vi "GoalieNormal.vi"(6 "atacando contra?":bool=TRUE, 7 "Stop?":bool=TRUE, 8 "Robot":T3={"id"=0, "function"=enum."Attacker", "x"=0.0, "y"=0.0, "orientation"=0.0, "v_tangent"=0.0, "v_normal"=0.0, "v_ang"=0.0, "kick_x"=0.0, "kick_z"=0.0, "dribble"=FALSE, "Timestamp"=timestamp(0 s since 1904-01-01), "estimatives"={"est_v_tangent"=0.0, "est_v_normal"=0.0, "est_vx"=0.0, "est_vy"=0.0, "Pos Robot Est"=[]}, "dest_x_kick"=0.0, "dest_y_kick"=0.0, "Gap Coord"=[], "States"=enum."GoToTangent", "Path "=[], "Path  Smooth"=[], "Dest"=[]}, 9 "AI Parameters":T1={"GotoKick"={"Dist do cone a frente"=150.0, "attacker farback"=1500.0, "Perto"=300.0, "min dist to kick"=150.0, "kick eps"=0.0, "Time to transition"=0.05}, "Attacker"={"CC chute"=0.09, "CC passe"=0.045, "Kick Force"=100.0, "ball-robot Kick"=200.0, "ball-robot Pass"=0.3, "drible\nAttk"=FALSE}, "Defender"={"D max"=1700.0, "Vel p/ robô av"=1000.0, "Kick Force"=100.0, "D atk-def"=0.0, "D farback"=0.0, "drible\ndef"=FALSE, "drible\ngoalie"=FALSE}, "Timeout"={"Field/v in x"=6.0, "Dist Robots"=300, "Dist up in y"=300}, "Pose Striker"={"dist"=200.0, "Numeric"=-4.0, "dist 2"=200.0, "drible\nstriker"=FALSE}, "Dist Stop"=300.0, "D ball out"=200, "D central gap "=150.0, "T pass"=0.0, "Force ++"=0.0, "range kick"=0.0, "Chute alto"=TRUE, "Marcador novo"=TRUE, "drible"=FALSE, "D drible"=300.0} {"D drible" format="%#_13g"; "D central gap" format="%#_13g"; "Dist Stop" format="%#_13g"; "Pose Striker"."Numeric" format="%#_13g"; "Defender"."Kick Force" format="%#_13g"; "Defender"."Vel p/ robô av" format="%#_13g"; "Attacker"."ball-robot Kick" format="%#_13g"; "Attacker"."Kick Force" format="%#_13g"; "Attacker"."CC passe" format="%#_13g"; "Attacker"."CC chute" format="%#_13g"; "GotoKick"."kick eps" format="%#_13g"; "GotoKick"."min dist to kick" format="%#_13g"; "GotoKick"."Perto" format="%#_13g"; "GotoKick"."attacker farback" format="%#_13g"; "GotoKick"."Dist do cone a frente" format="%#_13g"}, 10 "geometry":T2, 11 "IA Input":T8={"our_robots"=[], "enemy_robots"=[], "balls"=[], "geometry"={"line_width"=0, "field_length"=0, "field_width"=0, "boundary_width"=0, "referee_width"=0, "goal_width"=0, "goal_depth"=0, "goal_wall_width"=0, "center_circle_radius"=0, "defense_radius"=0, "defense_stretch"=0, "free_kick_from_defense_dist"=0, "penalty_spot_from_field_line_dist"=0, "penalty_line_from_spot_dist"=0}, "IA Judge"={"stage"="", "command"="", "our_goalie_id"=0.0, "enemy_goalie_id"=0.0, "command enum"=enum."Halt", "Time"=enum."Azul"}, "Received Timestamp"=timestamp(0 s since 1904-01-01), "Events"={"Touch"=FALSE, "Ball out"=FALSE, "id touch"=0.0, "Ball out of \nVision"=FALSE, "Ball inside \nGoalie area"=FALSE, "Robot not responding"=FALSE, "Robots responding status"=[1.0, 1.0, 1.0, 1.0, 1.0, 1.0], "Enemy Ball \nPossession"=FALSE, "Pass State"=FALSE, "id end of pass"=0.0, "Kick"=FALSE, "Id ini Possession"=0.0, "Ball Possesion"=FALSE, "Id Possesion"=0.0}}) -> (3 "output cluster":T3={"id"=0, "function"=enum."Attacker", "x"=0.0, "y"=0.0, "orientation"=0.0, "v_tangent"=0.0, "v_normal"=0.0, "v_ang"=0.0, "kick_x"=0.0, "kick_z"=0.0, "dribble"=FALSE, "Timestamp"=timestamp(0 s since 1904-01-01), "estimatives"={"est_v_tangent"=0.0, "est_v_normal"=0.0, "est_vx"=0.0, "est_vy"=0.0, "Pos Robot Est"=[]}, "dest_x_kick"=0.0, "dest_y_kick"=0.0, "Gap Coord"=[], "States"=enum."GoToTangent", "Path "=[], "Path  Smooth"=[], "Dest"=[]})   [LabVIEW 2017]
uses:
  Core/AI Input.ctl
  Core/AI Robot.ctl
  Functions Enum.ctl
  AttackerStates.ctl
  Path Planning/RRT/PathDests.ctl
  Path Planning/RRT/PathDest.ctl
  Core/AI Ball.ctl
  Core/Field Size.ctl
  Core/AI Judge.ctl
  Command Enum.ctl
  Util/Events/Events.ctl
  AI Parameters.ctl
  PersonalityEnum.ctl
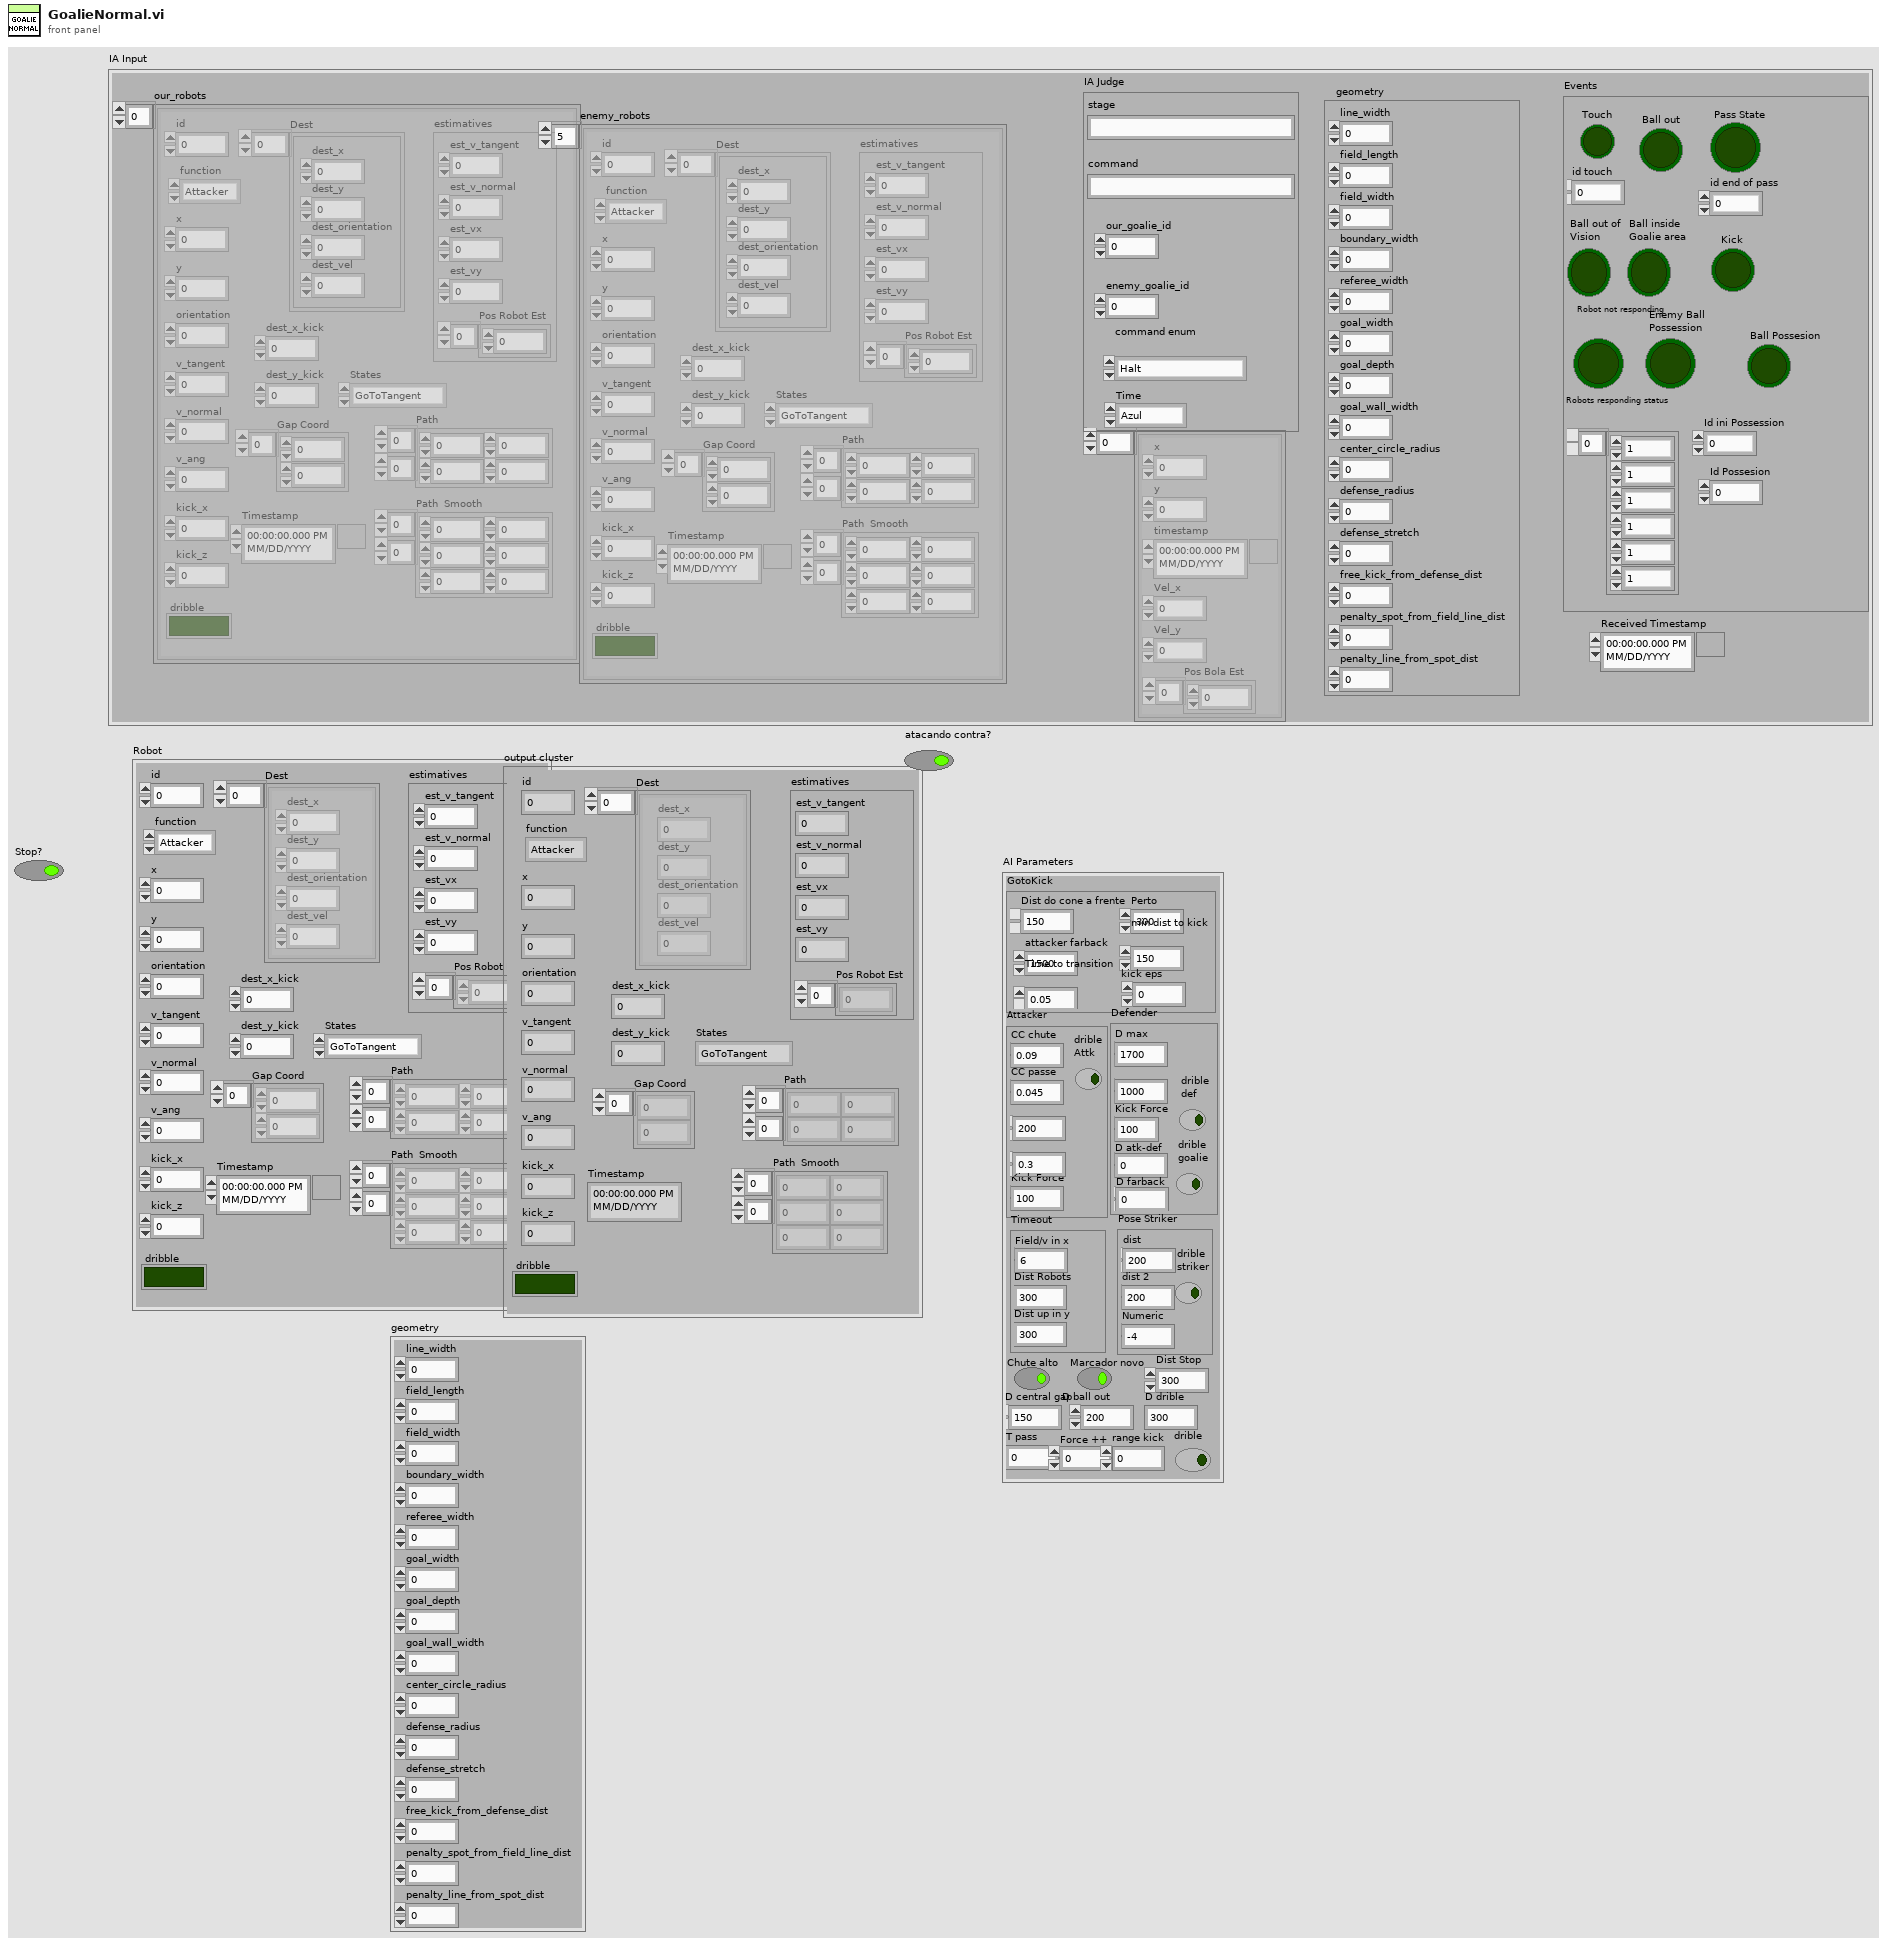
[diagram p1: front panel]
types:
  T1 = typedef "AI Parameters.ctl" = cluster{"GotoKick":cluster{"Dist do cone a frente":dbl, "attacker farback":dbl, "Perto":dbl, "min dist to kick":dbl, "kick eps":dbl, "Time to transition":dbl}, "Attacker":cluster{"CC chute":dbl, "CC passe":dbl, "Kick Force":dbl, "ball-robot Kick":dbl, "ball-robot Pass":dbl, "drible\nAttk":bool}, "Defender":cluster{"D max":dbl, "Vel p/ robô av":dbl, "Kick Force":dbl, "D atk-def":dbl, "D farback":dbl, "drible\ndef":bool, "drible\ngoalie":bool}, "Timeout":cluster{"Field/v in x":dbl, "Dist Robots":u32, "Dist up in y":u32}, "Pose Striker":cluster{"dist":dbl, "Numeric":dbl, "dist 2":dbl, "drible\nstriker":bool}, "Dist Stop":dbl, "D ball out":i32, "D central gap ":dbl, "T pass":dbl, "Force ++":dbl, "range kick":dbl, "Chute alto":bool, "Marcador novo":bool, "drible":bool, "D drible":dbl}
  T2 = typedef "Field Size.ctl" = cluster{"line_width":u32, "field_length":u32, "field_width":u32, "boundary_width":u32, "referee_width":u32, "goal_width":u32, "goal_depth":u32, "goal_wall_width":u32, "center_circle_radius":u32, "defense_radius":u32, "defense_stretch":u32, "free_kick_from_defense_dist":u32, "penalty_spot_from_field_line_dist":u32, "penalty_line_from_spot_dist":u32}
  T3 = typedef "AI Robot.ctl" = cluster{"id":u32, "function":T4, "x":dbl, "y":dbl, "orientation":dbl, "v_tangent":dbl, "v_normal":dbl, "v_ang":dbl, "kick_x":dbl, "kick_z":dbl, "dribble":bool, "Timestamp":timestamp, "estimatives":cluster{"est_v_tangent":dbl, "est_v_normal":dbl, "est_vx":dbl, "est_vy":dbl, "Pos Robot Est":dbl[]}, "dest_x_kick":dbl, "dest_y_kick":dbl, "Gap Coord":dbl[], "States":T5, "Path ":dbl[][], "Path  Smooth":dbl[][], "Dest":T6}
  T4 = typedef "Functions Enum.ctl" = enum16{"Attacker", "Goalie", "Defender", "Striker", "Goto 0", "Dummy", "Kicker", "ZigZag 0", "ZigZag 1", "ZigZag 2", "ZigZag 3", "ZigZag 4", "ZigZag 5", "ZigZag 6", "ZigZag 7", "ZigZag 8", ""}
  T5 = typedef "AttackerStates.ctl" = enum16{"Pass", "GoToTangent", "BallGetting", "GoToKick", ""}
  T6 = typedef "PathDests.ctl" = T7[]
  T7 = typedef "PathDest.ctl" = cluster{"dest_x":dbl, "dest_y":dbl, "dest_orientation":dbl, "dest_vel":dbl}
  T8 = typedef "AI Input.ctl" = cluster{"our_robots":T3[], "enemy_robots":T3[], "balls":T9[], "geometry":T2, "IA Judge":T10, "Received Timestamp":timestamp, "Events":T12}
  T9 = typedef "AI Ball.ctl" = cluster{"x":dbl, "y":dbl, "timestamp":timestamp, "Vel_x":dbl, "Vel_y":dbl, "Pos Bola Est":dbl[]}
  T10 = typedef "AI Judge.ctl" = cluster{"stage":string, "command":string, "our_goalie_id":dbl, "enemy_goalie_id":dbl, "command enum":T11, "Time":enum16{"Azul", "Amarelo"}}
  T11 = typedef "Command Enum.ctl" = enum16{"Halt", "Stop", "Force Start", "PKA Normal Start", "Prepare Kickoff Ally", "PKE Normal Start", "Prepare Kickoff Enemy", "Prepare Penalty Ally", "PPA Normal Start", "Prepare Penalty Enemy", "PPE Normal Start", "Direct Free Enemy", "Direct Free Ally", "Indirect Free Enemy", "Indirect Free Ally", "Timeout Enemy", "Timeout Ally", "Goal Enemy", "Goal Ally", "Ball Placement Enemy", "Ball Placement Ally", "Normal Half Time", "Extra Time Break", "Extra Half Time", "None", "Post Game"}
  T12 = typedef "Events.ctl" = cluster{"Touch":bool, "Ball out":bool, "id touch":dbl, "Ball out of \nVision":bool, "Ball inside \nGoalie area":bool, "Robot not responding":bool, "Robots responding status":dbl[], "Enemy Ball \nPossession":bool, "Pass State":bool, "id end of pass":dbl, "Kick":bool, "Id ini Possession":dbl, "Ball Possesion":bool, "Id Possesion":dbl}
  T13 = typedef "PersonalityEnum.ctl" = enum16{"Attacker", "Striker", "Defender", "Goalie"}
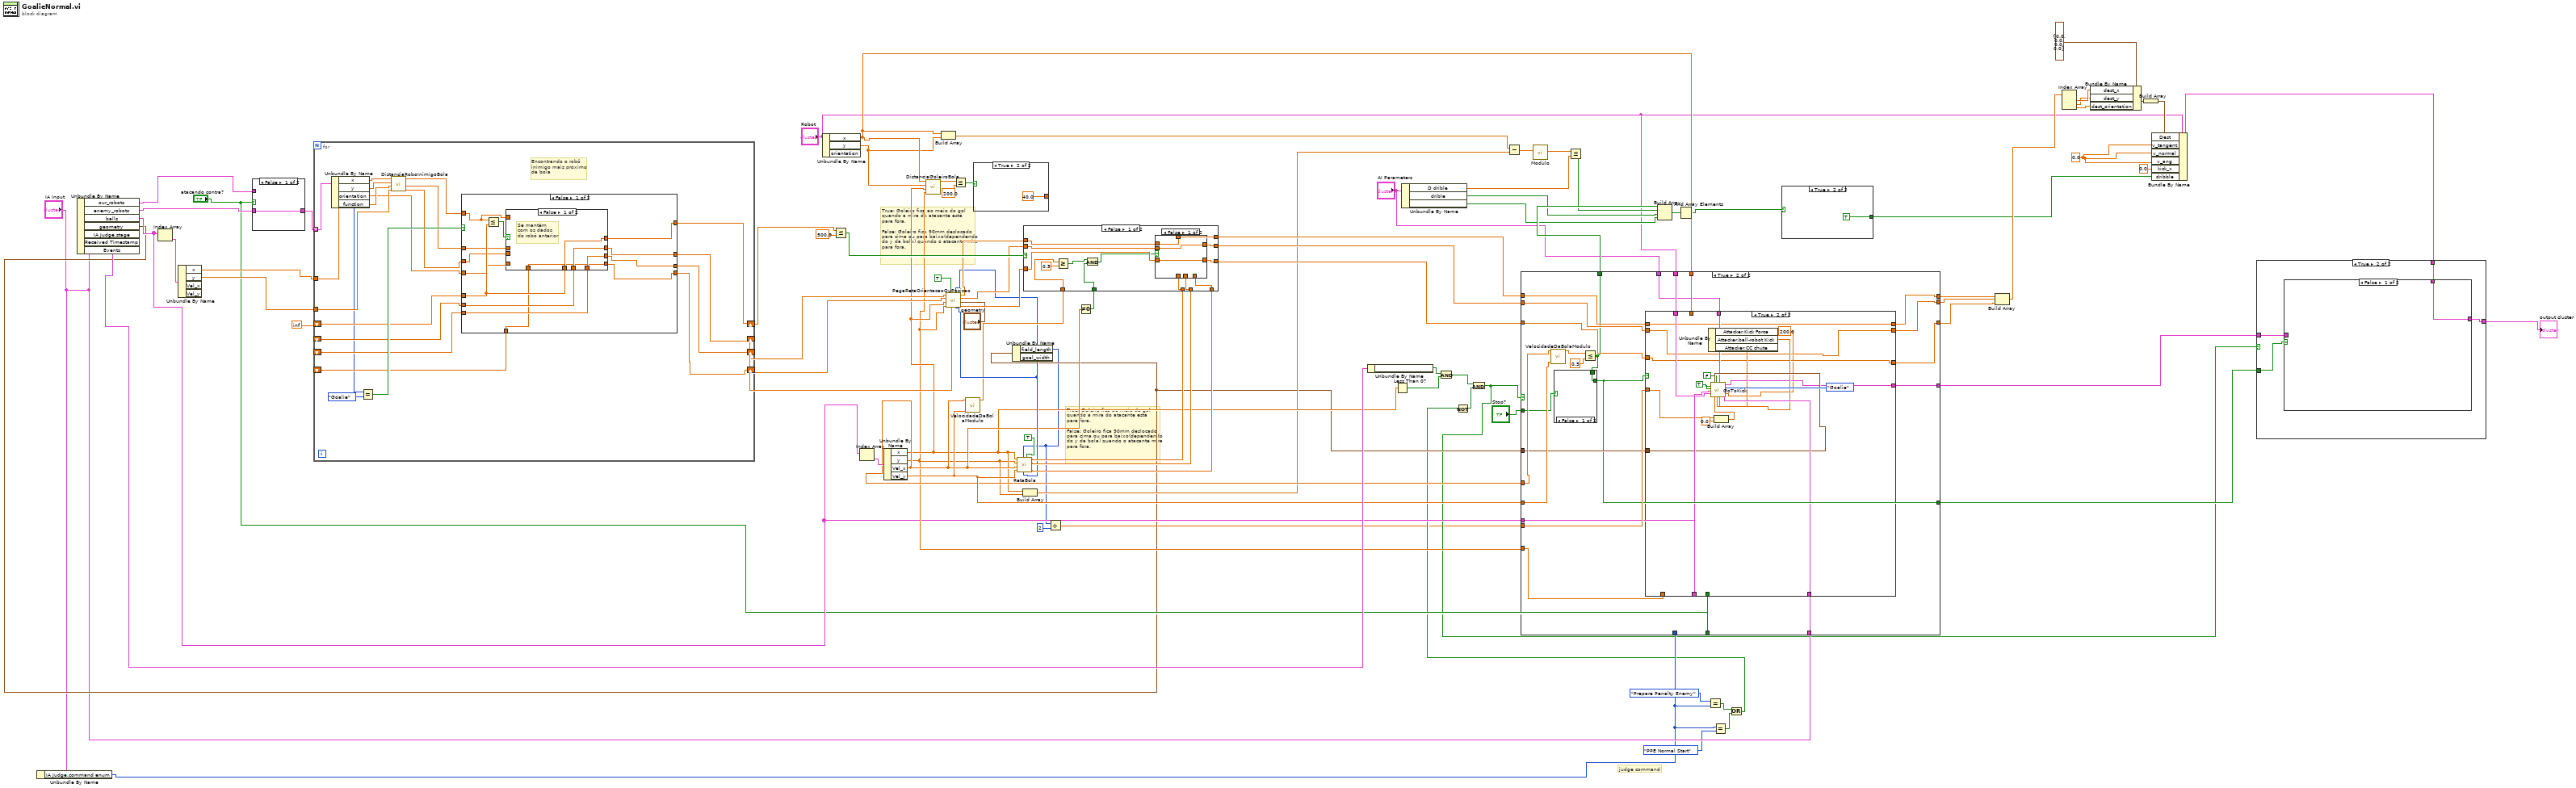
[diagram p0: block diagram]
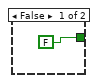
[diagram p4: hidden frame]
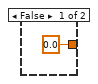
[diagram p6: hidden frame]
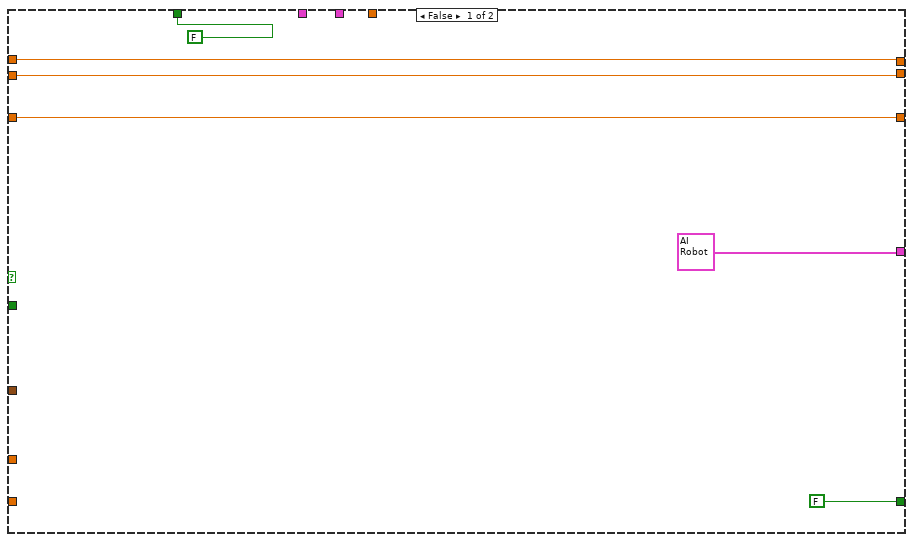
[diagram p7: hidden frame]
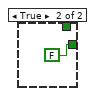
[diagram p8: hidden frame]
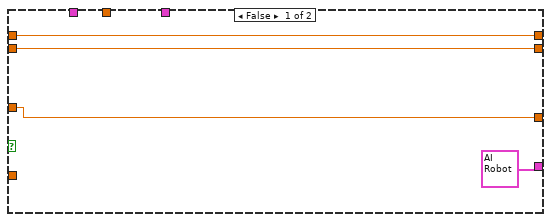
[diagram p9: hidden frame]
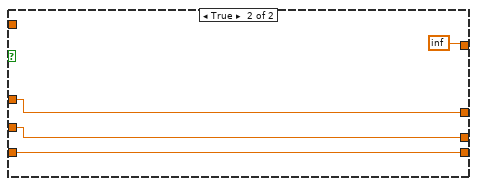
[diagram p13: hidden frame]
diagram:
  w41 = 0.0
  # "judge command"
  # "True: Goleiro fica ao meio do gol\nquando a mira do atacante está\npara fora.\n\nFalse: Goleiro fica 90mm deslocado\npara cima ou para baixo(dependendo\ndo y da bola) quando o atacante mira\npara fora."
  # "True: Goleiro fica ao meio do gol\nquando a mira do atacante está\npara fora.\n\nFalse: Goleiro fica 90mm deslocado\npara cima ou para baixo(dependendo\ndo y da bola) quando o atacante mira\npara fora."
  n1 = Unbundle By Name("IA Input") -> ("IA Judge.command enum"=w10:T11)
  n2 = Unbundle By Name("IA Input") -> ("our_robots"=w64:T3[], "enemy_robots"=w66:T3[], "balls"=w23:T9[], "geometry"=w20:T2, "Events"=w81:T12)  [unwired: 2 out]
  n3 = Index Array(array=w23) -> (element=w88:T9)  [unwired: 1 in]
  n4 = Unbundle By Name(w88) -> ("x"=w87:dbl, "y"=w86:dbl)  [unwired: 2 out]
  n5 = case shown="False" "atacando contra?" {
    tunnel: [w89 w90] -> w65
    tunnel: w66 -> [w89 _]
    tunnel: w64 -> [_ w90]
    frame False {
    }
    frame True {
    }
  }
  n6 = for {
    tunnel: w65 -> [w102] mode=indexing
    tunnel: w87 -> [w107]
    tunnel: w86 -> [w106]
    shift-right: [w104] -> w84
    shift-left: inf -> [w103]
    shift-right: [w100] -> w57
    shift-left: _ -> [w97]
    shift-right: [w98] -> w58
    shift-left: _ -> [w96]
    shift-right: [w94] -> w63
    shift-left: _ -> [w93]
    # "Encontrando o robô \ninimigo mais próximo\nda bola"
    n7 = Unbundle By Name(w102) -> ("x"=w109:dbl, "y"=w108:dbl, "orientation"=w95:dbl, "function"=w92:T4)
    n8 = Equal?(x=w92, y=Functions_Enum."Goalie") -> (x = y?=w110:bool)
    n9 = call "DistanciaRoboInimigoBola.vi"("Y bola"=w106, "X bola"=w107, "Y inimigo"=w108, "X inimigo"=w109) -> ("Y inimigo"=w99:dbl, "X inimigo"=w101:dbl, "Distância"=w105:dbl)  [unwired: 5 in]
    n10 = case shown="False" w110 {
      tunnel: [w122 inf] -> w104
      tunnel: w105 -> [w121 _]
      tunnel: w103 -> [w120 _]
      tunnel: w101 -> [w116 w135]
      tunnel: [w118 w135] -> w100
      tunnel: w99 -> [w115 w134]
      tunnel: [w112 w134] -> w98
      tunnel: w97 -> [w119 _]
      tunnel: w96 -> [w117 _]
      tunnel: w95 -> [w114 w133]
      tunnel: [w113 w133] -> w94
      tunnel: w93 -> [w111 _]
      frame False {
        n11 = Less Or Equal?(x=w121, y=w120) -> (x <= y?=w123:bool)
        n12 = case shown="False" w123 {
          tunnel: [w127 w131] -> w122
          tunnel: w121 -> [_ w131]
          tunnel: w120 -> [w127 _]
          tunnel: w119 -> [w126 _]
          tunnel: [w126 w130] -> w118
          tunnel: w117 -> [w125 _]
          tunnel: [w125 w129] -> w112
          tunnel: w116 -> [_ w130]
          tunnel: w115 -> [_ w129]
          tunnel: w114 -> [_ w128]
          tunnel: [w124 w128] -> w113
          tunnel: w111 -> [w124 _]
          frame False {
            # "Se mantém \ncom os dados\ndo robô anterior"
          }
          frame True {
            # "Fica com os\ndados do robô\natual"
          }
        }
      }
      frame True {
      }
    }
  }
  n13 = Unbundle By Name("Robot") -> ("x"=w40:dbl, "y"=w39:dbl)  [unwired: 1 out]
  n14 = Less Or Equal?(x=w84, y=500.0) -> (x <= y?=w82:bool)
  n15 = Index Array(array=w23) -> (element=w85:T9)  [unwired: 1 in]
  n16 = Unbundle By Name(w85) -> ("x"=w37:dbl, "y"=w36:dbl, "Vel_x"=w52:dbl, "Vel_y"=w53:dbl)
  n17 = call "DistanciaGoleiroBola.vi"("Y bola"=w36, "X bola"=w37, "Y goleiro"=w39, "X goleiro"=w40) -> ("Distância"=w74:dbl)  [unwired: 7 in]
  n18 = Build Array(w40, w39) -> (w38:dbl[])
  n19 = Less Or Equal?(x=w74, y=200.0) -> (x <= y?=w72:bool)
  n20 = call "VelocidadeDaBolaModulo.vi"("Vy bola"=w53, "Vx bola"=w52) -> ("Vel bola"=w54:dbl)  [unwired: 9 in]
  n21 = case shown="True" w72 {
    tunnel: [0.0 40.0] -> _
    frame False {
    }
    frame True {
    }
  }
  n22 = Unbundle By Name(w20) -> ("field_length"=w3:u32, "goal_width"=w62:u32)
  n23 = call "PegaRetaOrientacaoOuPosicao.vi"("Field Size 2"="geometry", "Goal Width"=w62, "Field Length"=w3, "Orientação inimigo"=w63, "Meio?"=TRUE, "Y bola"=w36, "X bola"=w37, "Y inimigo"=w58, "X inimigo"=w57) -> ("Orientação goleiro"=w59:dbl, "Y goleiro"=w60:dbl, "X goleiro"=w61:dbl)
  n24 = call "RetaBola.vi"("Meio?"=TRUE, "Goal Width"=w62, "Field Lenght"=w3, "Vy bola"=w53, "Vx bola"=w52, "Y bola"=w36, "X bola"=w37) -> ("Orientação"=w68:dbl, "Y goleiro"=w69:dbl, "X goleiro"=w70:dbl)  [unwired: 2 in]
  n25 = Build Array(w37, w36) -> (w35:dbl[])
  n26 = Divide(x=w3, y=u32 2) -> (x/y=w2:dbl)
  n27 = Not Equal To 0?(x=w52) -> (x != 0?=w51:bool)
  n28 = case shown="False" w82 {
    tunnel: [w149 w160] -> w80
    tunnel: w61 -> [w143 w160]
    tunnel: [w147 w159] -> w78
    tunnel: w60 -> [w142 w159]
    tunnel: [w144 w158] -> w76
    tunnel: w59 -> [w141 w158]
    tunnel: w70 -> [w148 _]
    tunnel: w69 -> [w146 _]
    tunnel: w68 -> [w145 _]
    tunnel: w54 -> [w150 _]
    tunnel: w51 -> [w139 _]
    frame False {
      n29 = Greater Or Equal?(x=w150, y=0.5) -> (x >= y?=w140:bool)
      n30 = And(x=w140, y=w139) -> (x .and. y?=w138:bool)
      n31 = case shown="False" w138 {
        tunnel: [w154 w157] -> w149
        tunnel: w148 -> [_ w157]
        tunnel: [w153 w156] -> w147
        tunnel: w146 -> [_ w156]
        tunnel: w145 -> [_ w155]
        tunnel: [w152 w155] -> w144
        tunnel: w143 -> [w154 _]
        tunnel: w142 -> [w153 _]
        tunnel: w141 -> [w152 _]
        frame False {
        }
        frame True {
        }
      }
    }
    frame True {
    }
  }
  n32 = Unbundle By Name(w81) -> ("Ball inside \nGoalie area"=w44:bool)
  n33 = Less Than 0?(x=w37) -> (x < 0?=w43:bool)
  n34 = Unbundle By Name("AI Parameters") -> ("D drible"=w32:dbl, "drible"=w28:bool, "Defender.drible\ngoalie"=w27:bool)
  n35 = And(x=w44, y=w43) -> (x .and. y?=w6:bool)
  n36 = Subtract(x=w38, y=w35) -> (x-y=w34:dbl[])
  n37 = call "Modulo.vi"("2D vector"=w34) -> ("Modulo"=w33:dbl)  [unwired: 10 in]
  n38 = Less Or Equal?(x=w33, y=w32) -> (x <= y?=w29:bool)
  n39 = Equal?(x=Command_Enum."Prepare Penalty Enemy", y=w10) -> (x = y?=w9:bool)
  n40 = Equal?(x=w10, y=Command_Enum."PPE Normal Start" ("x")) -> (x = y?=w8:bool)
  n41 = Or(x=w9, y=w8) -> (x .or. y?=w4:bool)
  n42 = Not(x=w4) -> (.not. x?=w7:bool)
  n43 = And(x=w6, y=w7) -> (x .and. y?=w5:bool)
  n44 = case shown="True" w5 {
    tunnel: w52 -> [_ w181]
    tunnel: w53 -> [_ w180]
    tunnel: [w166 w170] -> w79
    tunnel: w80 -> [w166 w188]
    tunnel: [w165 w169] -> w77
    tunnel: w78 -> [w165 w187]
    tunnel: [w164 w185] -> w75
    tunnel: w76 -> [w164 w186]
    tunnel: w2 -> [_ w184]
    tunnel: w36 -> [_ w183]
    tunnel: w40 -> [_ w182]
    tunnel: [FALSE w178] -> w30
    tunnel: "Stop?" -> [_ w177]
    tunnel: w23 -> [_ w176]
    tunnel: "Robot" -> [_ w175]
    tunnel: "atacando contra?" -> [_ w174]
    tunnel: "IA Input" -> [_ w173]
    tunnel: w20 -> [_ w172]
    tunnel: "AI Parameters" -> [_ w171]
    tunnel: [FALSE w168] -> w16
    tunnel: [T3 {"id"=0, "function"=enum."Attacker", "x"=0.0, "y"=0.0, "orientation"=0.0, "v_tangent"=0.0, "v_normal"=0.0, "v_ang"=0.0, "kick_x"=0.0, "kick_z"=0.0, "dribble"=FALSE, "Timestamp"=timestamp(0 s since 1904-01-01), "estimatives"={"est_v_tangent"=0.0, "est_v_normal"=0.0, "est_vx"=0.0, "est_vy"=0.0, "Pos Robot Est"=[]}, "dest_x_kick"=0.0, "dest_y_kick"=0.0, "Gap Coord"=[], "States"=enum."GoToTangent", "Path "=[], "Path  Smooth"=[], "Dest"=[]} ("Robot out") w167] -> w15
    tunnel: w10 -> [_ _]
    frame False {
    }
    frame True {
      n45 = call "VelocidadeDaBolaModulo.vi"("Vy bola"=w180, "Vx bola"=w181) -> ("Vel bola"=w179:dbl)  [unwired: 9 in]
      n46 = Less Or Equal?(x=w179, y=0.5) -> (x <= y?=w178:bool)
      n47 = case shown="False" w177 {
        tunnel: [w190 FALSE] -> w168
        tunnel: w178 -> [w190 _]
        frame False {
        }
        frame True {
        }
      }
      n48 = case shown="True" w168 {
        tunnel: w188 -> [w194 w201]
        tunnel: w187 -> [w193 w200]
        tunnel: w186 -> [w195 w199]
        tunnel: [w195 w199] -> w185
        tunnel: w184 -> [_ w209]
        tunnel: w183 -> [_ _]
        tunnel: w182 -> [_ _]
        tunnel: w176 -> [_ w211]
        tunnel: w175 -> [_ w210]
        tunnel: w174 -> [_ _]
        tunnel: w173 -> [_ w207]
        tunnel: w172 -> [_ w206]
        tunnel: w171 -> [_ w205]
        tunnel: [w194 w201] -> w170
        tunnel: [w193 w200] -> w169
        tunnel: [T3 {"id"=0, "function"=enum."Attacker", "x"=0.0, "y"=0.0, "orientation"=0.0, "v_tangent"=0.0, "v_normal"=0.0, "v_ang"=0.0, "kick_x"=0.0, "kick_z"=0.0, "dribble"=FALSE, "Timestamp"=timestamp(0 s since 1904-01-01), "estimatives"={"est_v_tangent"=0.0, "est_v_normal"=0.0, "est_vx"=0.0, "est_vy"=0.0, "Pos Robot Est"=[]}, "dest_x_kick"=0.0, "dest_y_kick"=0.0, "Gap Coord"=[], "States"=enum."GoToTangent", "Path "=[], "Path  Smooth"=[], "Dest"=[]} ("Robot out") w198] -> w167
        frame False {
        }
        frame True {
          w212 = TRUE ("goleiro?")
          n49 = Unbundle By Name(w205) -> ("Attacker.ball-robot Kick"=w204:dbl, "Attacker.CC chute"=w203:dbl)  [unwired: 1 out]
          n50 = Build Array(w209, 0.0 ("element")) -> (w208:dbl[])
          n51 = call "GoToKick.vi"("goleiro?"=w212, "Dribble"=w212, "balls"=w211, "Robot in in"=w210, "Field Size in"=w206, "Target"=w208, "Defender"=FALSE, "D ball - robot"=w204, "AI Parameters"=w205, "Cone de chute"=w203, "Personalidade"=PersonalityEnum."Goalie", "Kick Force"=200.0, "IA State Input in"=w207) -> ("Robot out"=w198:T3)  [unwired: 3 in, 3 out]
        }
      }
    }
  }
  n52 = Build Array(w30, w29, w28, w27) -> (w26:bool[])
  n53 = And Array Elements(Boolean array=w26) -> (logical AND=w25:bool)
  n54 = case shown="True" w25 {
    tunnel: [FALSE TRUE] -> w31
    frame False {
    }
    frame True {
    }
  }
  n55 = Build Array(w79, w77, w75) -> (w71:dbl[])
  n56 = Index Array(array=w71) -> (element #1=w49:dbl, element #2=w48:dbl, element #3=w47:dbl)  [unwired: 3 in]
  n57 = Bundle By Name(cluster=T7 {"dest_x"=0.0, "dest_y"=0.0, "dest_orientation"=0.0, "dest_vel"=0.0} ("element"), "dest_x"=w49, "dest_y"=w48, "dest_orientation"=w47) -> (w46:T7)
  n58 = Build Array(w46) -> (w45:T7[])
  n59 = Bundle By Name(cluster="Robot", "Dest"=w45, "v_tangent"=w41, "v_normal"=w41, "v_ang"=w41, "kick_x"=0.0, "dribble"=w31) -> (w17:T3)
  n60 = case shown="True" w5 {
    tunnel: [w216 w219] -> w18
    tunnel: w17 -> [w216 w218]
    tunnel: w16 -> [_ w220]
    tunnel: w15 -> [_ w217]
    frame False {
    }
    frame True {
      n61 = case shown="False" w220 {
        tunnel: [w221 w222] -> w219
        tunnel: w218 -> [w221 _]
        tunnel: w217 -> [_ w222]
        frame False {
        }
        frame True {
        }
      }
    }
  }
  "output cluster" <- w18
